vi "Menu Build File Item.vi"() -> (3 "Menu File Item":refnum<data-value>)   [LabVIEW 2018, in "LF2R IDE.lvlib" / "LF2R IDE.lvclass"]
uses:
  LF2R IDE.lvclass
  <userlib>/_MGI/Menu Building/MenuItem/MGI_MenuItem.lvclass
  Menu Item.ctl
  <userlib>/_MGI/Menu Building/MenuItem/MenuSeparatorItem/MGI_MenuSeparatorItem.lvclass
  C:/Program Files (x86)/National Instruments/LabVIEW 2018/user.lib/_MGI/Menu Building/MenuItem/MGI_MenuItem.lvclass
  <userlib>/_MGI/Menu Building/MenuItem/MenuItem.vi
  <userlib>/_MGI/Menu Building/MenuItem/MenuSeparatorItem/MenuSeparatorItem.vi
  <userlib>/_MGI/Menu Building/MenuItem/Write Sub-Menus.vi
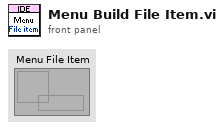
[diagram p1: front panel]
types:
  T1 = typedef "LF2R IDE.lvlib/LF2R IDE.lvclass/Menu Item.ctl" = enum16{"INVALID ITEM", "Open File", "Save File", "Exit", "Preferences"}
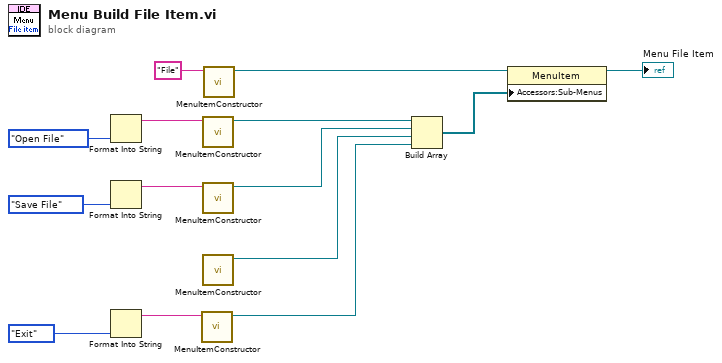
[diagram p0: block diagram]
diagram:
  n1 = Format Into String(Menu_Item."Open File" ("Menu item")) -> (resulting string=w7:string)  [unwired: 3 in, 1 out]
  n2 = Format Into String(Menu_Item."Save File" ("Menu item")) -> (resulting string=w4:string)  [unwired: 3 in, 1 out]
  n3 = Format Into String(Menu_Item."Exit" ("Menu item")) -> (resulting string=w5:string)  [unwired: 3 in, 1 out]
  n4 = call-poly <userlib>:"MenuItemConstructor.vi"("Text"=w5) -> ("MenuItem"=w10:refnum<data-value>)  [unwired: 9 in, 1 out]
  n5 = call-poly <userlib>:"MenuItemConstructor.vi"("Text"=w7) -> ("MenuItem"=w12:refnum<data-value>)  [unwired: 9 in, 1 out]
  n6 = call-poly <userlib>:"MenuItemConstructor.vi"("Text"=w4) -> ("MenuItem"=w2:refnum<data-value>)  [unwired: 9 in, 1 out]
  n7 = call-poly <userlib>:"MenuItemConstructor.vi"() -> ("MenuSeparatorItem"=w11:refnum<data-value>)  [unwired: 10 in, 1 out]
  n8 = call-poly <userlib>:"MenuItemConstructor.vi"("Text"="File") -> ("MenuItem"=w14:refnum<data-value>)  [unwired: 9 in, 1 out]
  n9 = Build Array(w12, w2, w11, w10) -> (w9:refnum<data-value>[])
  n10 = property class="MenuItem"(reference=w14, "Accessors:Sub-Menus"=w9) -> (reference out=→"Menu File Item":refnum<data-value>)  [unwired: 1 in, 1 out]
